vi "Remove Scan Engine Custom Device.vi"(8 "error in":errorcluster, 11 "scan engine custom device ref in":T1 format="%.0x") -> (0 "error out":errorcluster)   [LabVIEW 2017, in "Scan Engine Scripting.lvlib"]
doc: "Removes the Scan Engine and EtherCAT custom device."
uses:
  Scan Engine Scripting.lvlib
  <vilib>/NI Veristand/Custom Device API/Custom Device Item Ref.ctl
  Globals/Scan Engine GUIDs.vi
  Scan Engine Custom Device.lvlib
  <vilib>/NI Veristand/Custom Device API/Custom Device API.lvlib
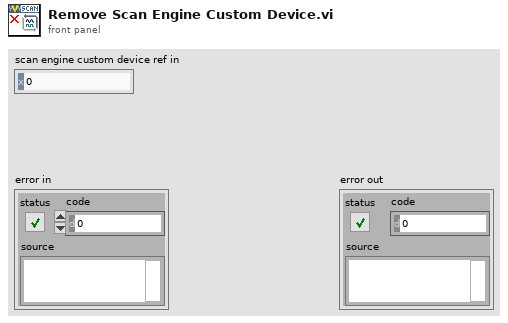
[diagram p1: front panel]
types:
  T1 = typedef "Custom Device API.lvlib/Custom Device Item Ref.ctl" = u64
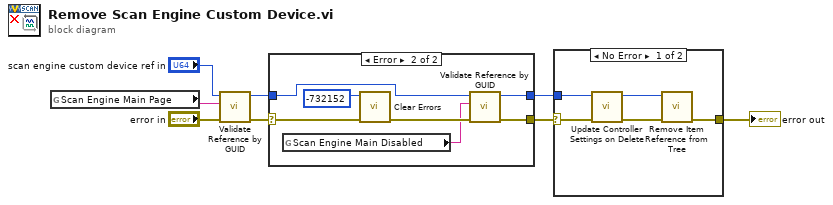
[diagram p0: block diagram]
diagram:
  n1 = global read "Scan Engine GUIDs.vi" "Scan Engine Main Page"() -> (w5:string)
  n2 = call "Validate Reference by GUID.vi"("error in"="error in", "GUID"=w5, "item in"="scan engine custom device ref in") -> ("error out"=w4:errorcluster, "item out"=w3:T1)  [unwired: 7 in]
  n3 = case shown="Error" w4 {
    selector: w4 -> [w9 w17]
    tunnel: w3 -> [w10 w14]
    tunnel: [w10 w12] -> w2
    tunnel: [w9 w11] -> w1
    frame No Error {
    }
    frame Error {
      n4 = global read "Scan Engine GUIDs.vi" "Scan Engine Main Disabled"() -> (w13:string)
      n5 = call <vilib>:"Clear Errors.vi"("error in (no error)"=w17, "specific error code to clear (0: all)"=-732152) -> ("error out"=w15:errorcluster)  [unwired: 4 in, 1 out]
      n6 = call "Validate Reference by GUID.vi"("error in"=w15, "GUID"=w13, "item in"=w14) -> ("error out"=w11:errorcluster, "item out"=w12:T1)  [unwired: 7 in]
    }
  }
  n7 = case shown="No Error" w1 {
    selector: w1 -> [w18 w23]
    tunnel: [w22 w23] -> w8
    tunnel: w2 -> [w21 _]
    frame No Error {
      n8 = call "Update Controller Settings on Delete.vi"("error in (no error)"=w18, "Item Ref in"=w21) -> ("error out"=w19:errorcluster, "Item Ref out"=w20:T1)  [unwired: 8 in]
      n9 = call "Remove Item Reference from Tree.vi"("error in"=w19, "item ref"=w20) -> ("error out"=w22:errorcluster)  [unwired: 8 in, 1 out]
    }
    frame Error {
    }
  }
  "error out" <- w8
